vi "SnesorHost.vi"() -> ()   [LabVIEW 2010]
uses:
  <vilib>/NXT/Subs/LVHSConnector.ctl
  <vilib>/NXT/Block Support/NXT_InputPort.ctl
  <vilib>/NXT/HiTechnic/HiTechnic Controls/HiTechnic Port.ctl
  <vilib>/NXT/NXTIO Xnodes/AddressXNode/NXTIOAddress.xnode
  <vilib>/NXT/Subs/MotorXNode.DC Motor Type.ctl
  <vilib>/NXT/Subs/MotorXNode.1DCMotor.ctl
  <vilib>/NXT/NXTIO Xnodes/NXTIOXNode/NXTIO.xnode
  <vilib>/NXT/HiTechnic/HiTechnic Read/HiTechnic EOPD Sensor Long.vi
  <vilib>/NXT/NXTIO Xnodes/NXTIONodeSubVIs/TETRIX IO Motor Status.vi
panel:
  out "Lift Encoder":i32
  out "Left Light":i16 caption="Scaled Value"
  out "EOPD Value":i16
  out "Right Light":i16 caption="Scaled Value"
  out "Direction (0-9)":i16
  in  "stop":bool
  out "Signal Strength (Array)":u8[](array[numeric])
  out "NXT":T1={"Hardware"="NXT", "Flattened String"=""}
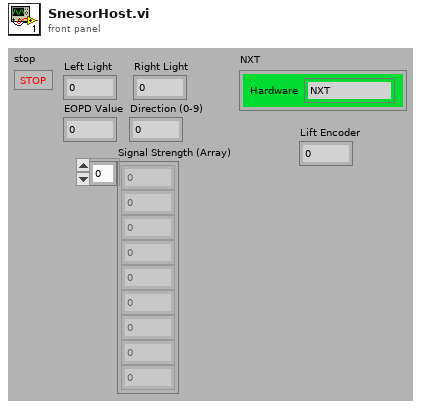
[diagram p1: front panel]
types:
  T1 = typedef "LVHSConnector.ctl" = cluster{"Hardware":string, "Flattened String":string}
  T2 = typedef "NXT_InputPort.ctl" = u8
  T3 = typedef "HiTechnic Port.ctl" = cluster{"Port":T2, "MUX Port":u8}
  T4 = cluster{"Direction (0-9)":i16, "Signal Strength (Array)":u8[]}
  T5 = typedef "MotorXNode.DC Motor Type.ctl" = enum16{"DC Motor"}
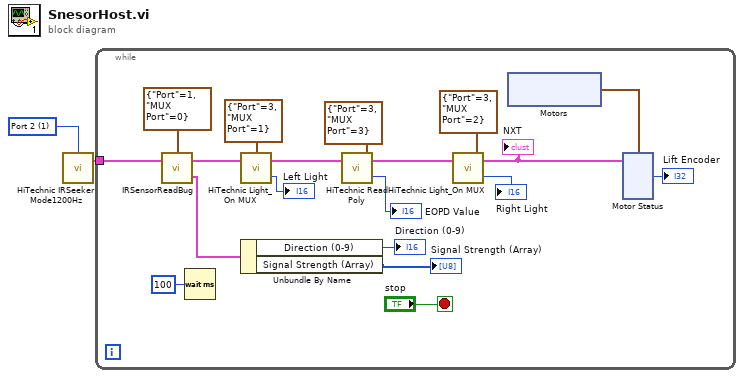
[diagram p0: block diagram]
diagram:
  w1 = T2 1 items=["Port 1", "Port 2", "Port 3", "Port 4"] ("Port")
  n1 = call <vilib>:"HiTechnic IRSeeker Mode1200Hz.vi"("Port"=w1) -> ("NXT"=w2:T1)  [unwired: 3 in]
  n2 = while {
    tunnel: w2 -> [w9]
    stop <- "stop" stop-if-true
    n3 = call "IRSensorReadBug.vi"("NXT 2"=w9, "Port/MUX"=T3 {"Port"=1, "MUX Port"=0}) -> ("All Info"=w7:T4, "NXT"=w8:T1)  [unwired: 1 in]
    n4 = Wait (ms)(milliseconds to wait=u32 100) -> ()  [unwired: 1 out]
    n5 = call <vilib>:"HiTechnic Light_On MUX.vi"("NXT"=w8, "Port/MUX"=T3 {"Port"=3, "MUX Port"=1}) -> ("Scaled Value"=→"Left Light":i16, "NXT"=w11:T1)  [unwired: 1 in]
    n6 = Unbundle By Name(w7) -> ("Direction (0-9)"=→"Direction (0-9)":i16, "Signal Strength (Array)"=→"Signal Strength (Array)":u8[])
    n7 = call-poly <vilib>:"HiTechnic Read Poly.vi"("NXT"=w11, "Port/MUX"=T3 {"Port"=3, "MUX Port"=3}) -> ("EOPD Value"=→"EOPD Value":i16, "NXT"=w10:T1)  [unwired: 1 in]
    n8 = call <vilib>:"HiTechnic Light_On MUX.vi"("NXT"=w10, "Port/MUX"=T3 {"Port"=3, "MUX Port"=2}) -> ("Scaled Value"=→"Right Light":i16, "NXT"=w3:T1)  [unwired: 1 in]
    "NXT" <- w3
    n9 = xnode "Motors"() -> ("DC Motor"=w5:cluster{"DC Motor":T5, "Address":i16})
    n10 = xnode "Motor Status"("Motors"=w5, "NXT"=w3) -> ("Position 1"=→"Lift Encoder":i32)  [unwired: 2 out]
  }
